vi "Create Notification.vi"(8 "error in (no error)":errorcluster, 9 "params":variant, 10 "method":string, 11 "Request":refnum<class "Request.lvclass">) -> (0 "error out":errorcluster, 2 "JSON Notificaiton":string, 3 "Request":refnum<class "Request.lvclass">)   [LabVIEW 2019, in "Request.lvclass"]
uses:
  Request.lvclass
  Request.lvclass/Request.ctl
  lv-venv/lv.lib/vi.lib/addons/_JKI.lib/Serialization/JSON/JKI JSON Serialization.lvlib
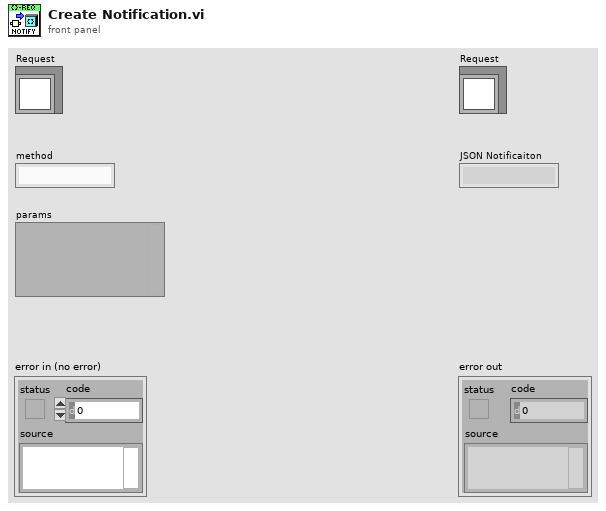
[diagram p1: front panel]
types:
  T1 = cluster{"jsonrpc":string, "method":string, "params":variant}
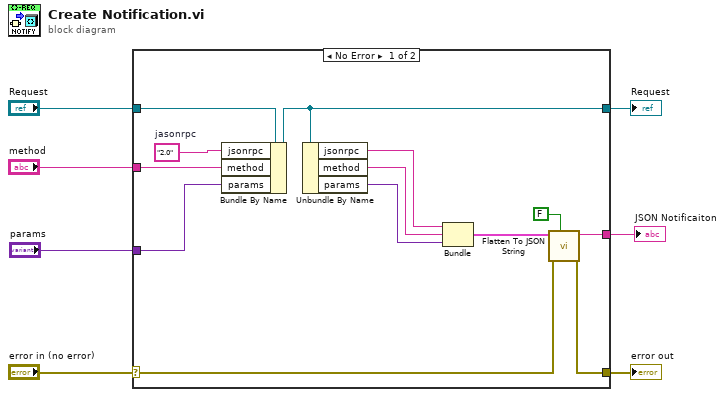
[diagram p0: block diagram]
diagram:
  n1 = case shown="No Error" "error in (no error)" {
    selector: "error in (no error)" -> [w19 w22]
    tunnel: [w18 w22] -> w6
    tunnel: [w11 w21] -> w4
    tunnel: "Request" -> [w20 w21]
    tunnel: "method" -> [w14 _]
    tunnel: "params" -> [w12 _]
    tunnel: [w16 _] -> w1
    frame No Error {
      w15 = "2.0"  # jasonrpc
      n2 = Bundle By Name(cluster=w20, "jsonrpc"=w15, "method"=w14, "params"=w12) -> (w11:refnum<class "Request.lvclass">)
      n3 = Unbundle By Name(w11) -> ("jsonrpc"=w10:string, "method"=w9:string, "params"=w8:variant)
      n4 = Bundle("jsonrpc"=w10, "method"=w9, "params"=w8) -> (w13:T1)  [unwired: 1 in]
      n5 = call "Flatten To JSON String.vi"("Multiline (T)"=FALSE, "error in (no error)"=w19, "Variant"=w13) -> ("error out"=w18:errorcluster, "JSON String"=w16:string)  [unwired: 7 in]
    }
    frame Error {
    }
  }
  "error out" <- w6
  "Request" <- w4
  "JSON Notificaiton" <- w1
